vi "Remove.vi"(8 "error in":errorcluster, 11 "Uno in":refnum<class "Uno.lvclass">) -> (0 "error out":errorcluster, 3 "Uno out":refnum<class "Uno.lvclass">)   [LabVIEW 2020, in "Uno.lvclass"]
uses:
  Uno.lvclass
  Uno.lvclass/Uno.ctl
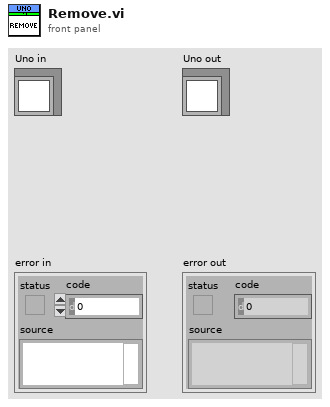
[diagram p1: front panel]
types:
  T1 = typedef "Uno.lvclass/Group Data.ctl" = cluster{"our positions":u8[][]}
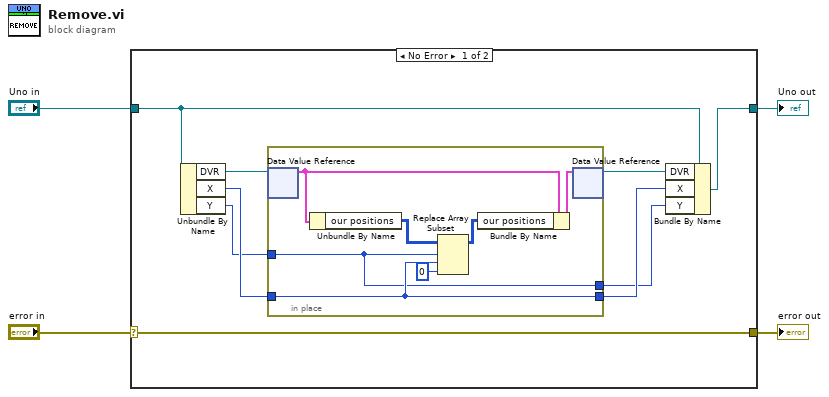
[diagram p0: block diagram]
diagram:
  n1 = case shown="No Error" "error in" {
    selector: "error in" -> [w13 w22]
    tunnel: [w13 w22] -> w3
    tunnel: [w11 w21] -> w1
    tunnel: "Uno in" -> [w12 w21]
    frame No Error {
      n2 = Unbundle By Name(w12) -> ("DVR"=w9:refnum<data-value>, "X"=w6:i32, "Y"=w5:i32)
      n3 = in-place {
        in-place-border: w5 -> [w15]
        in-place-border: w6 -> [w16]
        in-place-border: [w16] -> w8
        in-place-border: [w15] -> w7
        n4 = in-place-dvr #1(w9) -> (w20:T1)  [unwired: 1 out]
        n5 = Unbundle By Name(w20) -> ("our positions"=w18:u8[][])
        n6 = Replace Array Subset(array=w18, new element=u8 0 ("new element/subarray"), index (row)=w15, index (col)=w16) -> (w17:u8[][])
        n7 = Bundle By Name(cluster=w20, "our positions"=w17) -> (w19:T1)
        n8 = in-place-dvr #1(w19) -> (w10:refnum<data-value>)  [unwired: 1 out]
      }
      n9 = Bundle By Name(cluster=w12, "DVR"=w10, "X"=w8, "Y"=w7) -> (w11:refnum<class "Uno.lvclass">)
    }
    frame Error {
    }
  }
  "error out" <- w3
  "Uno out" <- w1
